vi "Add Linked List to Parent.vi"(6 "Insertion Index":i32=-1, 7 "Parent ID":string, 8 "error in (no error)":errorcluster, 10 "Linked List ID":string, 11 "Linked List Ref":refnum<data-value>) -> (0 "error out":errorcluster, 3 "Linked List Ref out":refnum<data-value>)   [LabVIEW 2019, in "Linked Lists.lvlib" / "Linked List Ref.lvclass"]
uses:
  <vilib>/gpm_packages/@cs/linked-list/Source/Linked List/Linked List Ref/Linked List Ref.lvclass
  <vilib>/gpm_packages/@cs/linked-list/Source/Linked List/ILinkedList/ILinked List.lvclass
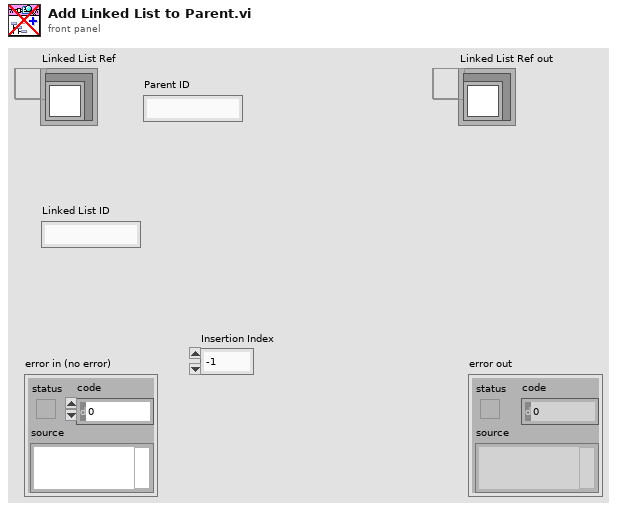
[diagram p1: front panel]
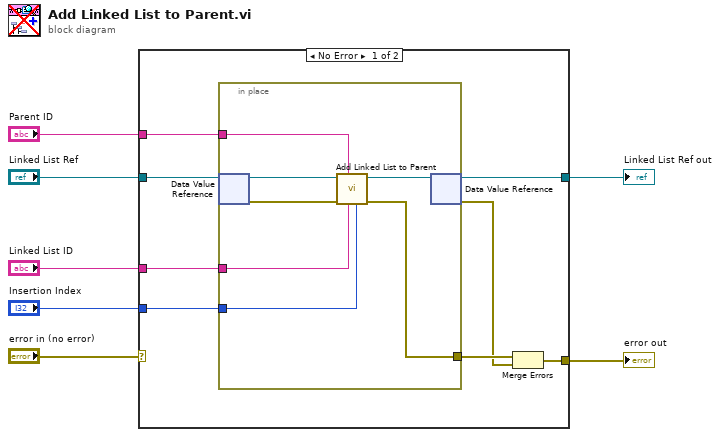
[diagram p0: block diagram]
diagram:
  n1 = case shown="No Error" "error in (no error)" {
    selector: "error in (no error)" -> [_ w24]
    tunnel: [w9 w24] -> w6
    tunnel: "Linked List Ref" -> [w14 w23]
    tunnel: [w13 w23] -> w4
    tunnel: "Parent ID" -> [w12 _]
    tunnel: "Linked List ID" -> [w11 _]
    tunnel: "Insertion Index" -> [w10 _]
    frame No Error {
      n2 = in-place {
        in-place-border: [w18] -> w15
        in-place-border: w12 -> [w20]
        in-place-border: w11 -> [w17]
        in-place-border: w10 -> [w16]
        n3 = in-place-dvr #1(w14) -> (w22:refnum<class "ILinked List.lvclass">, w19:errorcluster)
        n4 = call-dynamic "Add Linked List to Parent.vi"("Insertion Index"=w16, "Linked List ID"=w17, "Parent ID"=w20, "error in (no error)"=w19, "ILinked List in"=w22) -> ("error out"=w18:errorcluster, "ILinked List out"=w21:refnum<class "ILinked List.lvclass">)  [unwired: 5 in]
        n5 = in-place-dvr #1(w21) -> (w13:refnum<data-value>, w8:errorcluster)
      }
      n6 = Merge Errors(w15, w8) -> (w9:errorcluster)
    }
    frame Error {
    }
  }
  "error out" <- w6
  "Linked List Ref out" <- w4
